vi "HV Edit PMT File.vi"(9 "Append Single PMT?":bool, 11 "Rewrite PMT File Here\nPMT                  V1                     V2                    V3                     V4":string[][](array[string])) -> ()   [LabVIEW 2018]
uses:
  <vilib>/Utility/file.llb/Write Delimited Spreadsheet (string).vi
  HV_QMH/HV QMH.lvlib
panel:
  in  "?":T1(tab)
  in  "Append Single PMT to File Here\nPMT                  V1                     V2                    V3                     V4":string[](array[string])
  out "Current PMT File\nPMT                  V1                     V2                    V3                     V4":string[][](array[string])
  out "Number of PMTs":i32
  in  "Close":bool
  in  "Apply":bool
  # "Use the top set of scroll arrows next to each table to change the row being viewed"
  # "Use the top set of scroll arrows next to each table\nto change the row being viewed"
  # "This vi is used to edit the file that holds the PMT numbers and the voltages used for testing of each PMT.\n\nThe vi must be running before changes are made. If this has been opened via the HV Automation Demo application or the Main.vi, this should already be running.\n\nOn the \"Edit PMT File\" tab, there are two ways of editing the file.\n\nThe first way is rewriting the entire file. To do this, use the table labelled \"Rewrite PMT File\" here and fill in the PMT numbers and the respective voltages.\nMake sure the \"Append Single PMT?\" button is deselected (no green light) .\nPress the \"Apply\" button to apply the changes.\nThe new PMT file will be displayed in the \"Updated PMT File\" table.\n\nThe second way is to append one PMT to the file at a time.\nTo do this, select the \"Append Single PMT?\" button so that a green light is displayed.\nEnter the PMT number and its voltages into the \"Append Single PMT to File Here\" box.\nPress the \"Apply\" button.\n\nWhen finished, press the \"CLOSE\" button. This stops the vi and closes it down."
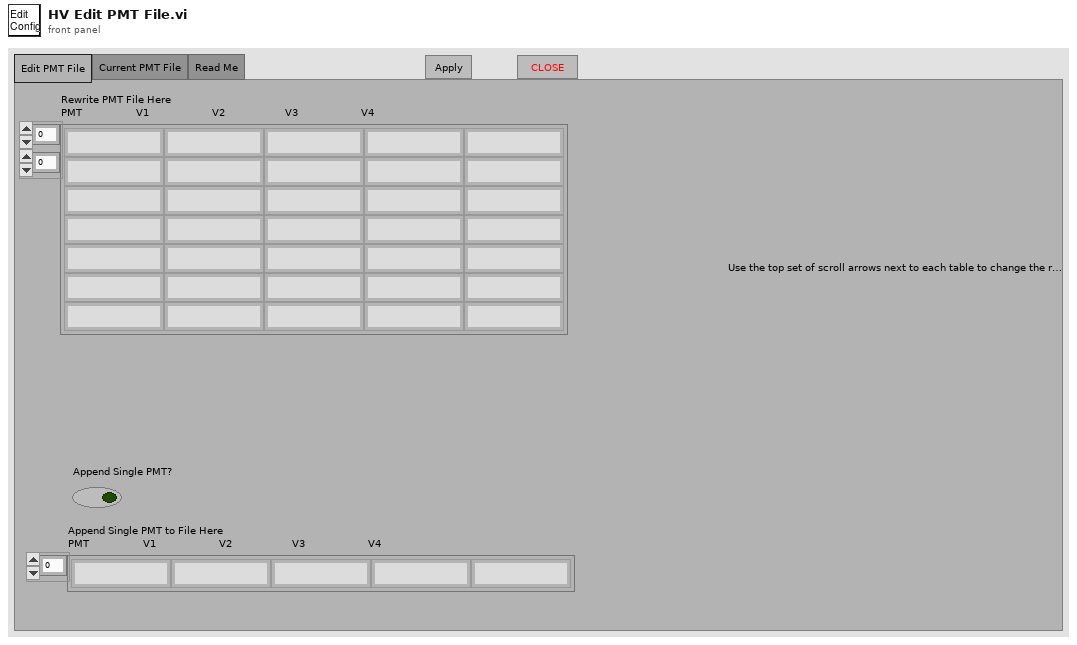
[diagram p1: front panel]
types:
  T1 = enum32{"Edit PMT File", "Current PMT File", "Read Me"}
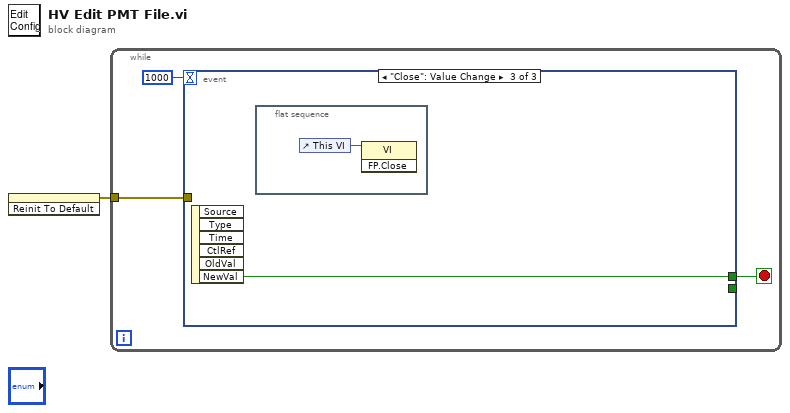
[diagram p0: block diagram]
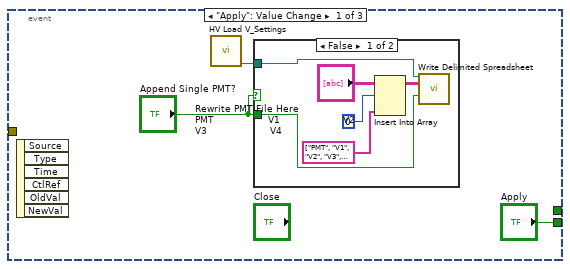
[diagram p2: hidden frame]
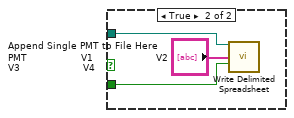
[diagram p3: hidden frame]
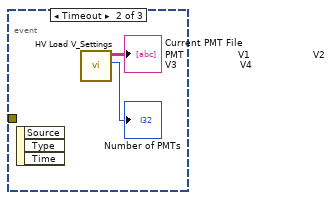
[diagram p4: hidden frame]
diagram:
  n1 = invoke on="Apply" class="Bool" method="Reinit To Default"() -> (error out=w1:errorcluster)  [unwired: 3 in, 2 out]
  n2 = while {
    tunnel: w1 -> [w4]
    stop <- w3 stop-if-true
    n3 = event shown="[2] \"Close\": Value Change" {
      selector: _ -> [_ _ _]
      dyn-events: _ -> [_ _ _]
      timeout: 1000 -> [_ _ _]
      tunnel: ["Apply" _ _] -> _
      tunnel: w4 -> [_ _ _]
      tunnel: [_ _ w19] -> w3
      event "Apply": Value Change {
        n4 = event-data() -> ()  [unwired: 1 in, 6 out]
        n5 = call "HV Load V_Settings.vi"() -> ("appended path"=w6:path)  [unwired: 9 in, 2 out]
        n6 = case shown="False" "Append Single PMT?" {
          tunnel: "Append Single PMT?" -> [w10 w16]
          tunnel: w6 -> [w8 w15]
          frame False {
            n7 = Insert Into Array(array="Rewrite PMT File Here\nPMT                  V1                     V2                    V3                     V4", index (row)=0, new element=string[] ["PMT", "V1", "V2", "V3", "V4"] ("new element/subarray")) -> (w9:string[][])  [unwired: 1 in]
            n8 = call-poly <vilib>:"Write Delimited Spreadsheet.vi"("file path (dialog if empty)"=w8, "2D data"=w9, "append to file? (new file:F)"=w10) -> ()  [unwired: 11 in, 2 out]
          }
          frame True {
            n9 = call-poly <vilib>:"Write Delimited Spreadsheet.vi"("file path (dialog if empty)"=w15, "1D data"="Append Single PMT to File Here\nPMT                  V1                     V2                    V3                     V4", "append to file? (new file:F)"=w16) -> ()  [unwired: 11 in, 2 out]
          }
        }
      }
      event Timeout {
        n10 = event-data() -> ()  [unwired: 1 in, 3 out]
        n11 = call "HV Load V_Settings.vi"() -> ("Number of PMTs"=→"Number of PMTs":i32, "V_Settings"=→"Current PMT File\nPMT                  V1                     V2                    V3                     V4":string[][])  [unwired: 9 in, 1 out]
      }
      event "Close": Value Change {
        n12 = event-data() -> ("NewVal"=w19:bool)  [unwired: 1 in, 5 out]
        n13 = flat-sequence {
          frame #0 {
            n14 = control-ref of="This VI"() -> (w20:refnum<vi>)
            n15 = invoke class="VI" method="FP.Close"(reference=w20) -> ()  [unwired: 2 in, 3 out]
          }
        }
      }
    }
  }
